vi "replaceSingleQuotes.vi"(8 "error in (no error)":errorcluster, 10 "XMLIn":string, 11 "AttributeReader in":refnum<class "XMLAttributeParser.lvclass">) -> (0 "error out":errorcluster, 2 "DoubleQuoteXML":string, 3 "AttributeReader out":refnum<class "XMLAttributeParser.lvclass">)   [LabVIEW 2014, in "XML.lvlib" / "XMLAttributeParser.lvclass"]
doc: "This VI simply finds any instance of single quotes and replaces it with double quotes."
uses:
  <userlib>/Common/XML/XMLAttributeParser/XMLAttributeParser.lvclass
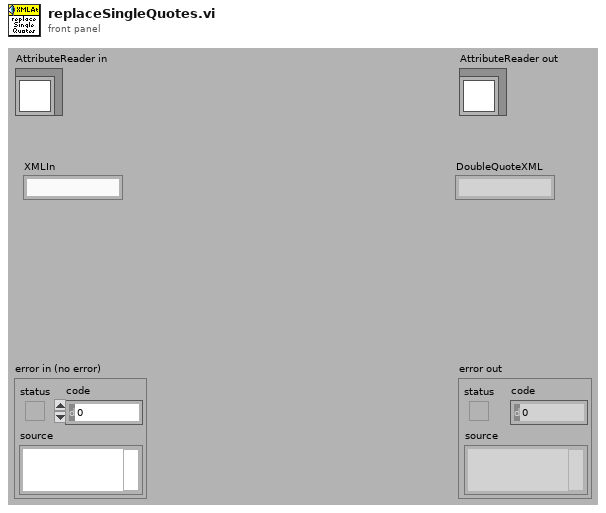
[diagram p1: front panel]
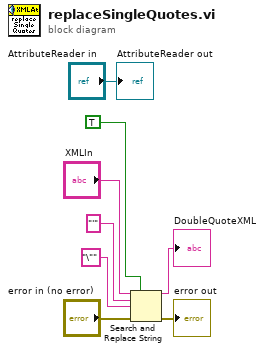
[diagram p0: block diagram]
diagram:
  n1 = Search and Replace String(replace all?=TRUE, input string="XMLIn", search string="'", replace string="\"" ("search string"), error in="error in (no error)") -> (result string=→"DoubleQuoteXML":string, error out=→"error out":errorcluster)  [unwired: 3 in, 2 out]
  "AttributeReader out" <- "AttributeReader in"
